vi "调用对话框设置参数.vi"() -> ()   [LabVIEW 2017]
uses:
  <vilib>/measure/NI_MABase.lvlib
panel:
  in  "退出程序":bool
  in  "停止按钮":bool
  in  "设置参数":bool
  out "波形图":waveform(dbl)(graph)
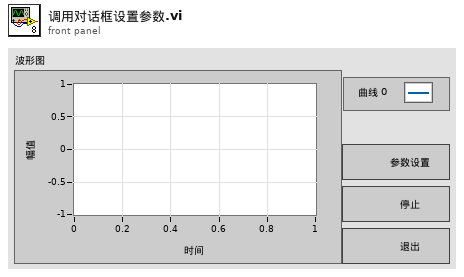
[diagram p1: front panel]
types:
  T1 = cluster{"frequency":dbl, "amplitude":dbl, "phase":dbl, "sampling info":cluster{"Fs":dbl, "#s":dbl}, "signal type":u16}
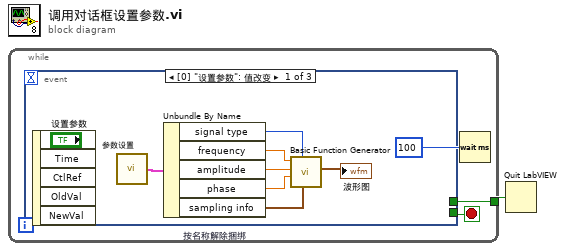
[diagram p0: block diagram]
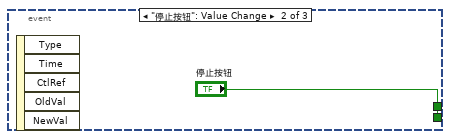
[diagram p2: hidden frame]
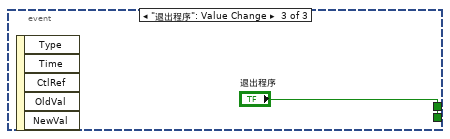
[diagram p3: hidden frame]
diagram:
  n1 = while {
    tunnel: [w2] -> w1
    stop <- w4 stop-if-true
    n2 = event shown="[0] \"设置参数\": 值改变" {
      selector: _ -> [_ _ _]
      dyn-events: _ -> [_ _ _]
      timeout: _ -> [_ _ _]
      tunnel: [_ "停止按钮" "退出程序"] -> w4
      tunnel: [_ _ "退出程序"] -> w2
      event "设置参数": Value Change {
        n3 = event-data() -> ()  [unwired: 1 in, 5 out]
        n4 = call "参数设置.vi"() -> ("设置完成的参数"=w11:T1)
        n5 = Unbundle By Name "按名称解除捆绑"(w11) -> ("signal type"=w9:u16, "frequency"=w8:dbl, "amplitude"=w7:dbl, "phase"=w6:dbl, "sampling info"=w5:cluster{"Fs":dbl, "#s":dbl})
        n6 = call <vilib>:"Basic Function Generator.vi"("sampling info"=w5, "signal type"=w9, "phase"=w6, "amplitude"=w7, "frequency"=w8) -> ("signal out"=→"波形图":waveform(dbl))  [unwired: 4 in, 2 out]
      }
      event "停止按钮": Value Change {
        n7 = event-data() -> ()  [unwired: 1 in, 5 out]
      }
      event "退出程序": Value Change {
        n8 = event-data() -> ()  [unwired: 1 in, 5 out]
      }
    }
    n9 = Wait (ms)(milliseconds to wait=u32 100 ("等待时间（毫秒）")) -> ()  [unwired: 1 out]
  }
  n10 = Quit LabVIEW(quit? (T)=w1) -> ()
